vi "_Config Rx FIFO.vi"(8 "error in (no error)":errorcluster, 9 "Requested Depth":u32=20480, 10 "Channel Number":u32, 11 "Refnum in":T1) -> (0 "error out":errorcluster, 3 "Refnum out":T1)   [LabVIEW 2020, in "985x Support Addon Engine.lvlib"]
uses:
  985x Support Addon Engine.lvlib
  Types/FPGA Refnum.ctl
  <vilib>/rvi/interface/common/niFpgaWaitOnOcc.vi
  <vilib>/Utility/error.llb/Error Cluster From Error Code.vi
  <vilib>/rvi/interface/nirviMethod/nirviMethod.xnode
  <vilib>/FPGAPlugInAG/Dynamic/niLvFpga_ConfigureFifo_Dynamic.vi
  <vilib>/rvi/errors/niLvFpgaMergeErrorWithErrorCode.vi
  <vilib>/FPGAPlugInAG/Dynamic/niLvFpga_StartFifo_Dynamic.vi
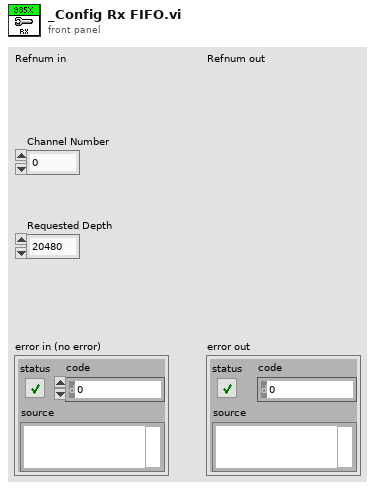
[diagram p1: front panel]
types:
  T1 = typedef "985x Support Addon Engine.lvlib/FPGA Refnum.ctl" = refnum<k20>
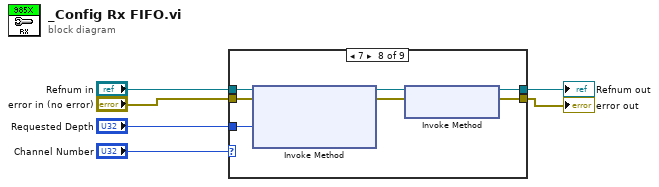
[diagram p0: block diagram]
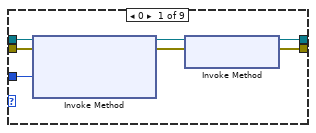
[diagram p2: hidden frame]
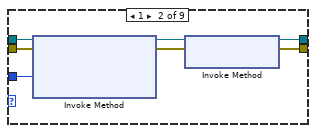
[diagram p3: hidden frame]
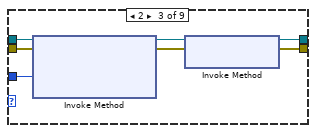
[diagram p4: hidden frame]
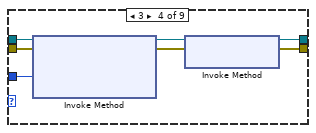
[diagram p5: hidden frame]
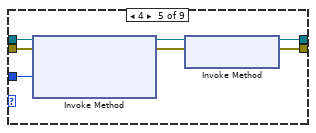
[diagram p6: hidden frame]
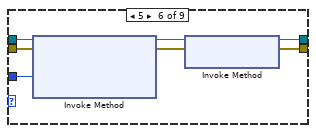
[diagram p7: hidden frame]
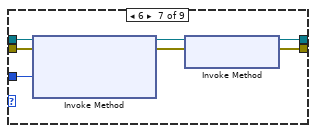
[diagram p8: hidden frame]
diagram:
  n1 = case shown="7" "Channel Number" {
    tunnel: "Refnum in" -> [w13 w20 w27 w34 w41 w48 w55 w62 w64]
    tunnel: "error in (no error)" -> [w12 w19 w26 w33 w40 w47 w54 w61 w63]
    tunnel: "Requested Depth" -> [w9 w16 w23 w30 w37 w44 w51 w58 _]
    tunnel: [w8 w15 w22 w29 w36 w43 w50 w57 w64] -> w5
    tunnel: [w7 w14 w21 w28 w35 w42 w49 w56 w63] -> w6
    frame 0 {
      n2 = xnode "Invoke Method"("FPGA VI Reference In"=w13, "error in"=w12, "Requested Depth"=w9) -> ("FPGA VI Reference Out"=w11:T1, "error out"=w10:errorcluster)  [unwired: 1 out]
      n3 = xnode "Invoke Method"("FPGA VI Reference In"=w11, "error in"=w10) -> ("FPGA VI Reference Out"=w8:T1, "error out"=w7:errorcluster)
    }
    frame 1 {
      n4 = xnode "Invoke Method"("FPGA VI Reference In"=w20, "error in"=w19, "Requested Depth"=w16) -> ("FPGA VI Reference Out"=w18:T1, "error out"=w17:errorcluster)  [unwired: 1 out]
      n5 = xnode "Invoke Method"("FPGA VI Reference In"=w18, "error in"=w17) -> ("FPGA VI Reference Out"=w15:T1, "error out"=w14:errorcluster)
    }
    frame 2 {
      n6 = xnode "Invoke Method"("FPGA VI Reference In"=w27, "error in"=w26, "Requested Depth"=w23) -> ("FPGA VI Reference Out"=w25:T1, "error out"=w24:errorcluster)  [unwired: 1 out]
      n7 = xnode "Invoke Method"("FPGA VI Reference In"=w25, "error in"=w24) -> ("FPGA VI Reference Out"=w22:T1, "error out"=w21:errorcluster)
    }
    frame 3 {
      n8 = xnode "Invoke Method"("FPGA VI Reference In"=w34, "error in"=w33, "Requested Depth"=w30) -> ("FPGA VI Reference Out"=w32:T1, "error out"=w31:errorcluster)  [unwired: 1 out]
      n9 = xnode "Invoke Method"("FPGA VI Reference In"=w32, "error in"=w31) -> ("FPGA VI Reference Out"=w29:T1, "error out"=w28:errorcluster)
    }
    frame 4 {
      n10 = xnode "Invoke Method"("FPGA VI Reference In"=w41, "error in"=w40, "Requested Depth"=w37) -> ("FPGA VI Reference Out"=w39:T1, "error out"=w38:errorcluster)  [unwired: 1 out]
      n11 = xnode "Invoke Method"("FPGA VI Reference In"=w39, "error in"=w38) -> ("FPGA VI Reference Out"=w36:T1, "error out"=w35:errorcluster)
    }
    frame 5 {
      n12 = xnode "Invoke Method"("FPGA VI Reference In"=w48, "error in"=w47, "Requested Depth"=w44) -> ("FPGA VI Reference Out"=w46:T1, "error out"=w45:errorcluster)  [unwired: 1 out]
      n13 = xnode "Invoke Method"("FPGA VI Reference In"=w46, "error in"=w45) -> ("FPGA VI Reference Out"=w43:T1, "error out"=w42:errorcluster)
    }
    frame 6 {
      n14 = xnode "Invoke Method"("FPGA VI Reference In"=w55, "error in"=w54, "Requested Depth"=w51) -> ("FPGA VI Reference Out"=w53:T1, "error out"=w52:errorcluster)  [unwired: 1 out]
      n15 = xnode "Invoke Method"("FPGA VI Reference In"=w53, "error in"=w52) -> ("FPGA VI Reference Out"=w50:T1, "error out"=w49:errorcluster)
    }
    frame 7 {
      n16 = xnode "Invoke Method"("FPGA VI Reference In"=w62, "error in"=w61, "Requested Depth"=w58) -> ("FPGA VI Reference Out"=w60:T1, "error out"=w59:errorcluster)  [unwired: 1 out]
      n17 = xnode "Invoke Method"("FPGA VI Reference In"=w60, "error in"=w59) -> ("FPGA VI Reference Out"=w57:T1, "error out"=w56:errorcluster)
    }
    frame Default {
    }
  }
  "error out" <- w6
  "Refnum out" <- w5
